vi "PicoScope2000aExampleBlockMSO.vi"() -> ()   [LabVIEW 2010]
doc: "ps2000a API Block Capture example"
uses:
  shared/PicoBuffers.ctl
  <vilib>/Waveform/DWDTOps.llb/DWDT Analog to Digital.vi
  shared/Buffer and Transfer Settings.ctl
  shared/Acquisition Settings.ctl
  PicoScope2000aLib/PicoScope2000aAnalogChannelSettings.ctl
  PicoScope2000aLib/PicoScope2000aDigitalChannelSettings.ctl
panel:
  out "Pico 2000a Units":string
  in  "roundFaster":bool=TRUE
  in  "timeIntervalRequested":dbl format="%#6_6p"
  in  "Write to TDMS":bool
  out "Properties Panel":T1 {"Max Total Capture Time Available (sec)" format="%.3p"; "Sample Frequency" format="%.3p"; "Sample Internal" format="%.3p"; "Max Samples Available" format="%.3p"; "Total Capture Time (sec)" format="%.3p"}
  in  "Port 0 Settings":T2={"Enabled"=FALSE, "Logic Level"=9830} {"Logic Level" items=["1.5V TTL"=9830, "2.5V CMOS"=16383]}
  in  "Channel A Settings":T3={"Enabled"=TRUE, "Coupling"=1, "Range"=6, "Analogue Offset"=0.0} {"Analogue Offset" format="%#_6p"; "Range" items=["20 mV"=1, "50 mV"=2, "100 mV"=3, "200 mV"=4, "500 mV"=5, "1 V"=6, "2 V"=7, "5 V"=8, "10 V"=9, "20 V"=10]; "Coupling" items=["AC", "DC"]}
  out "Device Info":T4={"Driver Version"="0", "USB Version"="0", "Hardware"="1", "Variant"="0", "Batch and Serial"="0", "Cal Date"="0", "Kernel Version"="0", "Digital HW Version"="0", "Analogue HW Version"="0", "Firmware 1"="0", "Firmware 2"="0", "MSO"=FALSE, "Number of Channels"=0}
  out "overflow":i16 format="%06b"
  in  "Apply Settings":bool
  in  "Trigger Settings":T5={"Trigger Enabled"=FALSE, "Trigger Source"=enum."Channel A", "Trigger Threshold (volts)"=0.0, "Trigger Direction"=2, "Trigger Delay (samples)"=0, "Auto Trigger Time (ms)"=1000} {"Trigger Direction" items=["Rising"=2, "Falling"=3]}
  out "error out":errorcluster
  in  "Data file":path=path "PicoScope2000aExampleBlock Data"
  in  "Buffer and Transfer Settings":T6={"startIndex"=0, "Samples"=32000, "Down Sample Ratio"=1, "Down-Sample Mode"=0} {"Down-Sample Mode" items=["RAW none"=2147483648, "None"=0, "Aggregate"=1, "Decimate"=2, "Average"=4]; "Down Sample Ratio" step=1; "Samples" format="%_6p"}
  in  "Acquisition Settings":T7={"preTriggerSamples"=0, "postTriggerSamples"=32000, "timebase"=0} {"postTriggerSamples" format="%_6p"; "preTriggerSamples" format="%_6p"}
  out "Port 0":digitalwaveform(graph)={"t0"=timestamp(0 s since 1904-01-01), "dt"=8e-09, "Y"={"transitions"=[], "data"=[]}}
  in  "stop":bool
  out "Analog Channels":cluster{i32, sgl, "Data":dbl[]}[](graph)
  in  "Serial Number":string
  in  "Use Serial Number":bool
  in  "error in (no error)":errorcluster
  # "Bit 0 = ChA"
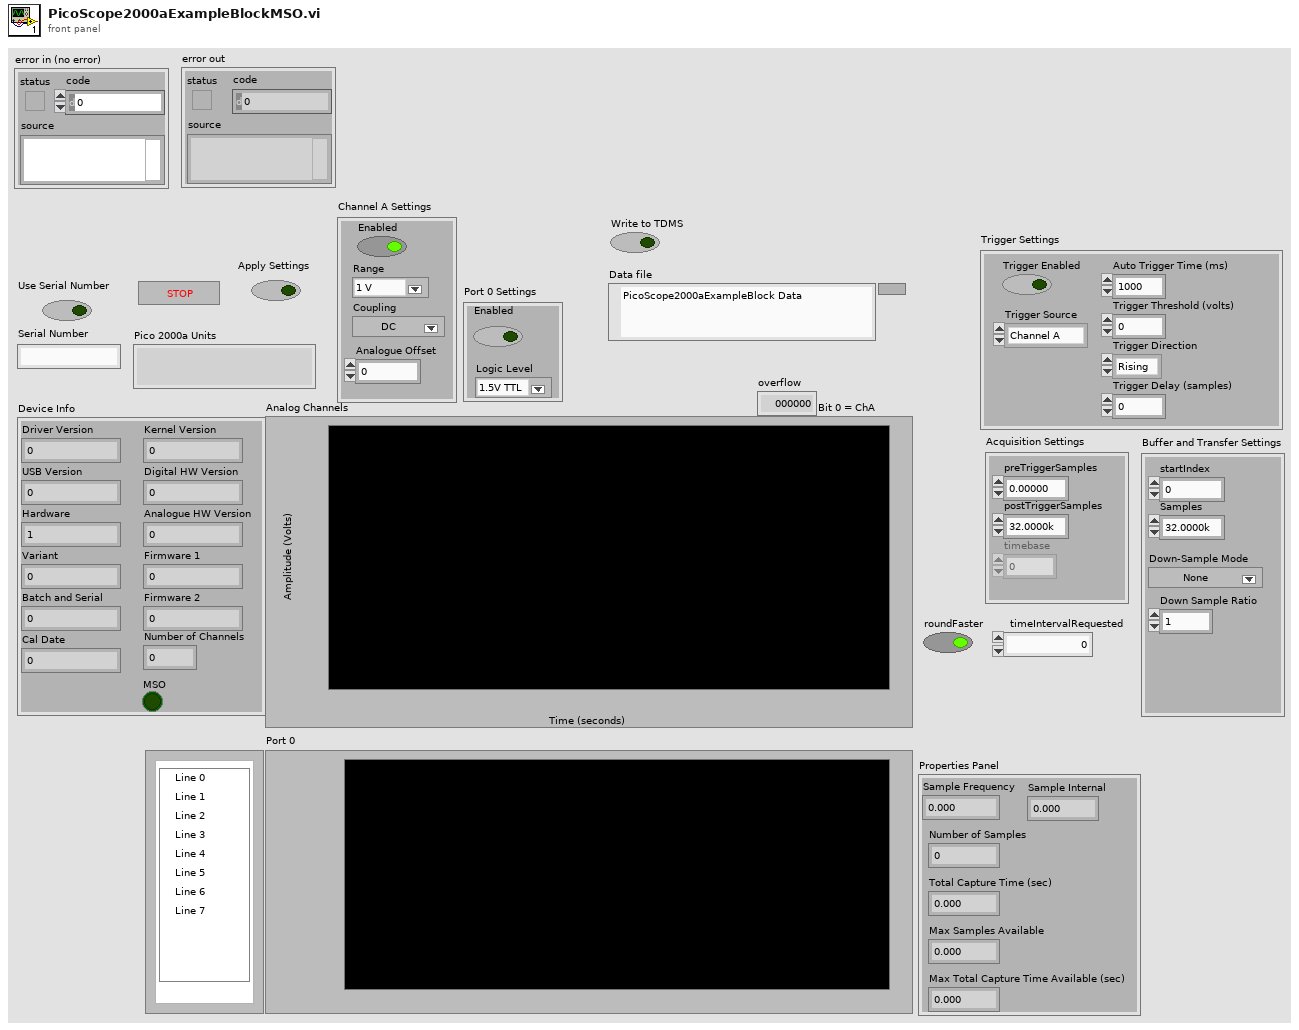
[diagram p1: front panel]
types:
  T1 = cluster{"Sample Frequency":sgl, "Sample Internal":sgl, "Max Samples Available":i32, "Number of Samples":u32, "Total Capture Time (sec) ":sgl, "Max Total Capture Time Available (sec)":sgl}
  T2 = typedef "PicoScope2000aDigitalChannelSettings.ctl" = cluster{"Enabled":bool, "Logic Level":i16}
  T3 = typedef "PicoScope2000aAnalogChannelSettings.ctl" = cluster{"Enabled":bool, "Coupling":i16, "Range":u32, "Analogue Offset":sgl}
  T4 = cluster{"Driver Version":string, "USB Version":string, "Hardware":string, "Variant":string, "Batch and Serial":string, "Cal Date":string, "Kernel Version":string, "Digital HW Version":string, "Analogue HW Version":string, "Firmware 1":string, "Firmware 2":string, "MSO":bool, "Number of Channels":i16}
  T5 = cluster{"Trigger Enabled":bool, "Trigger Source":enum16{"Channel A", "Channel B", "Channel C", "Channel D", "Ext."}, "Trigger Threshold (volts)":dbl, "Trigger Direction":u16, "Trigger Delay (samples)":u32, "Auto Trigger Time (ms)":i16}
  T6 = typedef "Buffer and Transfer Settings.ctl" = cluster{"startIndex":u64, "Samples":u64, "Down Sample Ratio":u64, "Down-Sample Mode":u32}
  T7 = typedef "Acquisition Settings.ctl" = cluster{"preTriggerSamples":u64, "postTriggerSamples":u64, "timebase":u32}
  T8 = typedef "PicoBuffers.ctl" = cluster{"Max Buffer Pointers":u64[][][], "Min Buffer Pointers":u64[][][], "StreamingDataInfo":cluster{"Channel":u32, "Down-Sample Mode":u32, "PICO_DATA_TYPE":enum32{"PICO_INT8_T", "PICO_INT16_T", "PICO_INT32_T", "PICO_UINT32_T", "PICO_INT64_T", ""}, "Samples":i32, "bufferIndex":u64, "startIndex":i32, "overflow":i16}[][]}
  T9 = enum16{"open", "open or create", "create or replace", "create", "open (read-only)"}
  T10 = cluster{"Channel A Buffer":i16[], "Channel B Buffer":i16[], "Channel C Buffer":i16[], "Channel D Buffer":i16[], "Channel E Buffer":i16[], "Channel F Buffer":i16[], "Channel G Buffer":i16[], "Channel H Buffer":i16[], "Port 0 Buffer":i16[], "Port 1 Buffer":i16[]}[]
  T11 = cluster{"Channel A Buffer":i16[], "Channel B Buffer":i16[], "Channel C Buffer":i16[], "Channel D Buffer":i16[], "Channel E Buffer":i16[], "Channel F Buffer":i16[], "Channel G Buffer":i16[], "Channel H Buffer":i16[], "Port 0 Buffer":i16[], "Port 1 Buffer":i16[]}
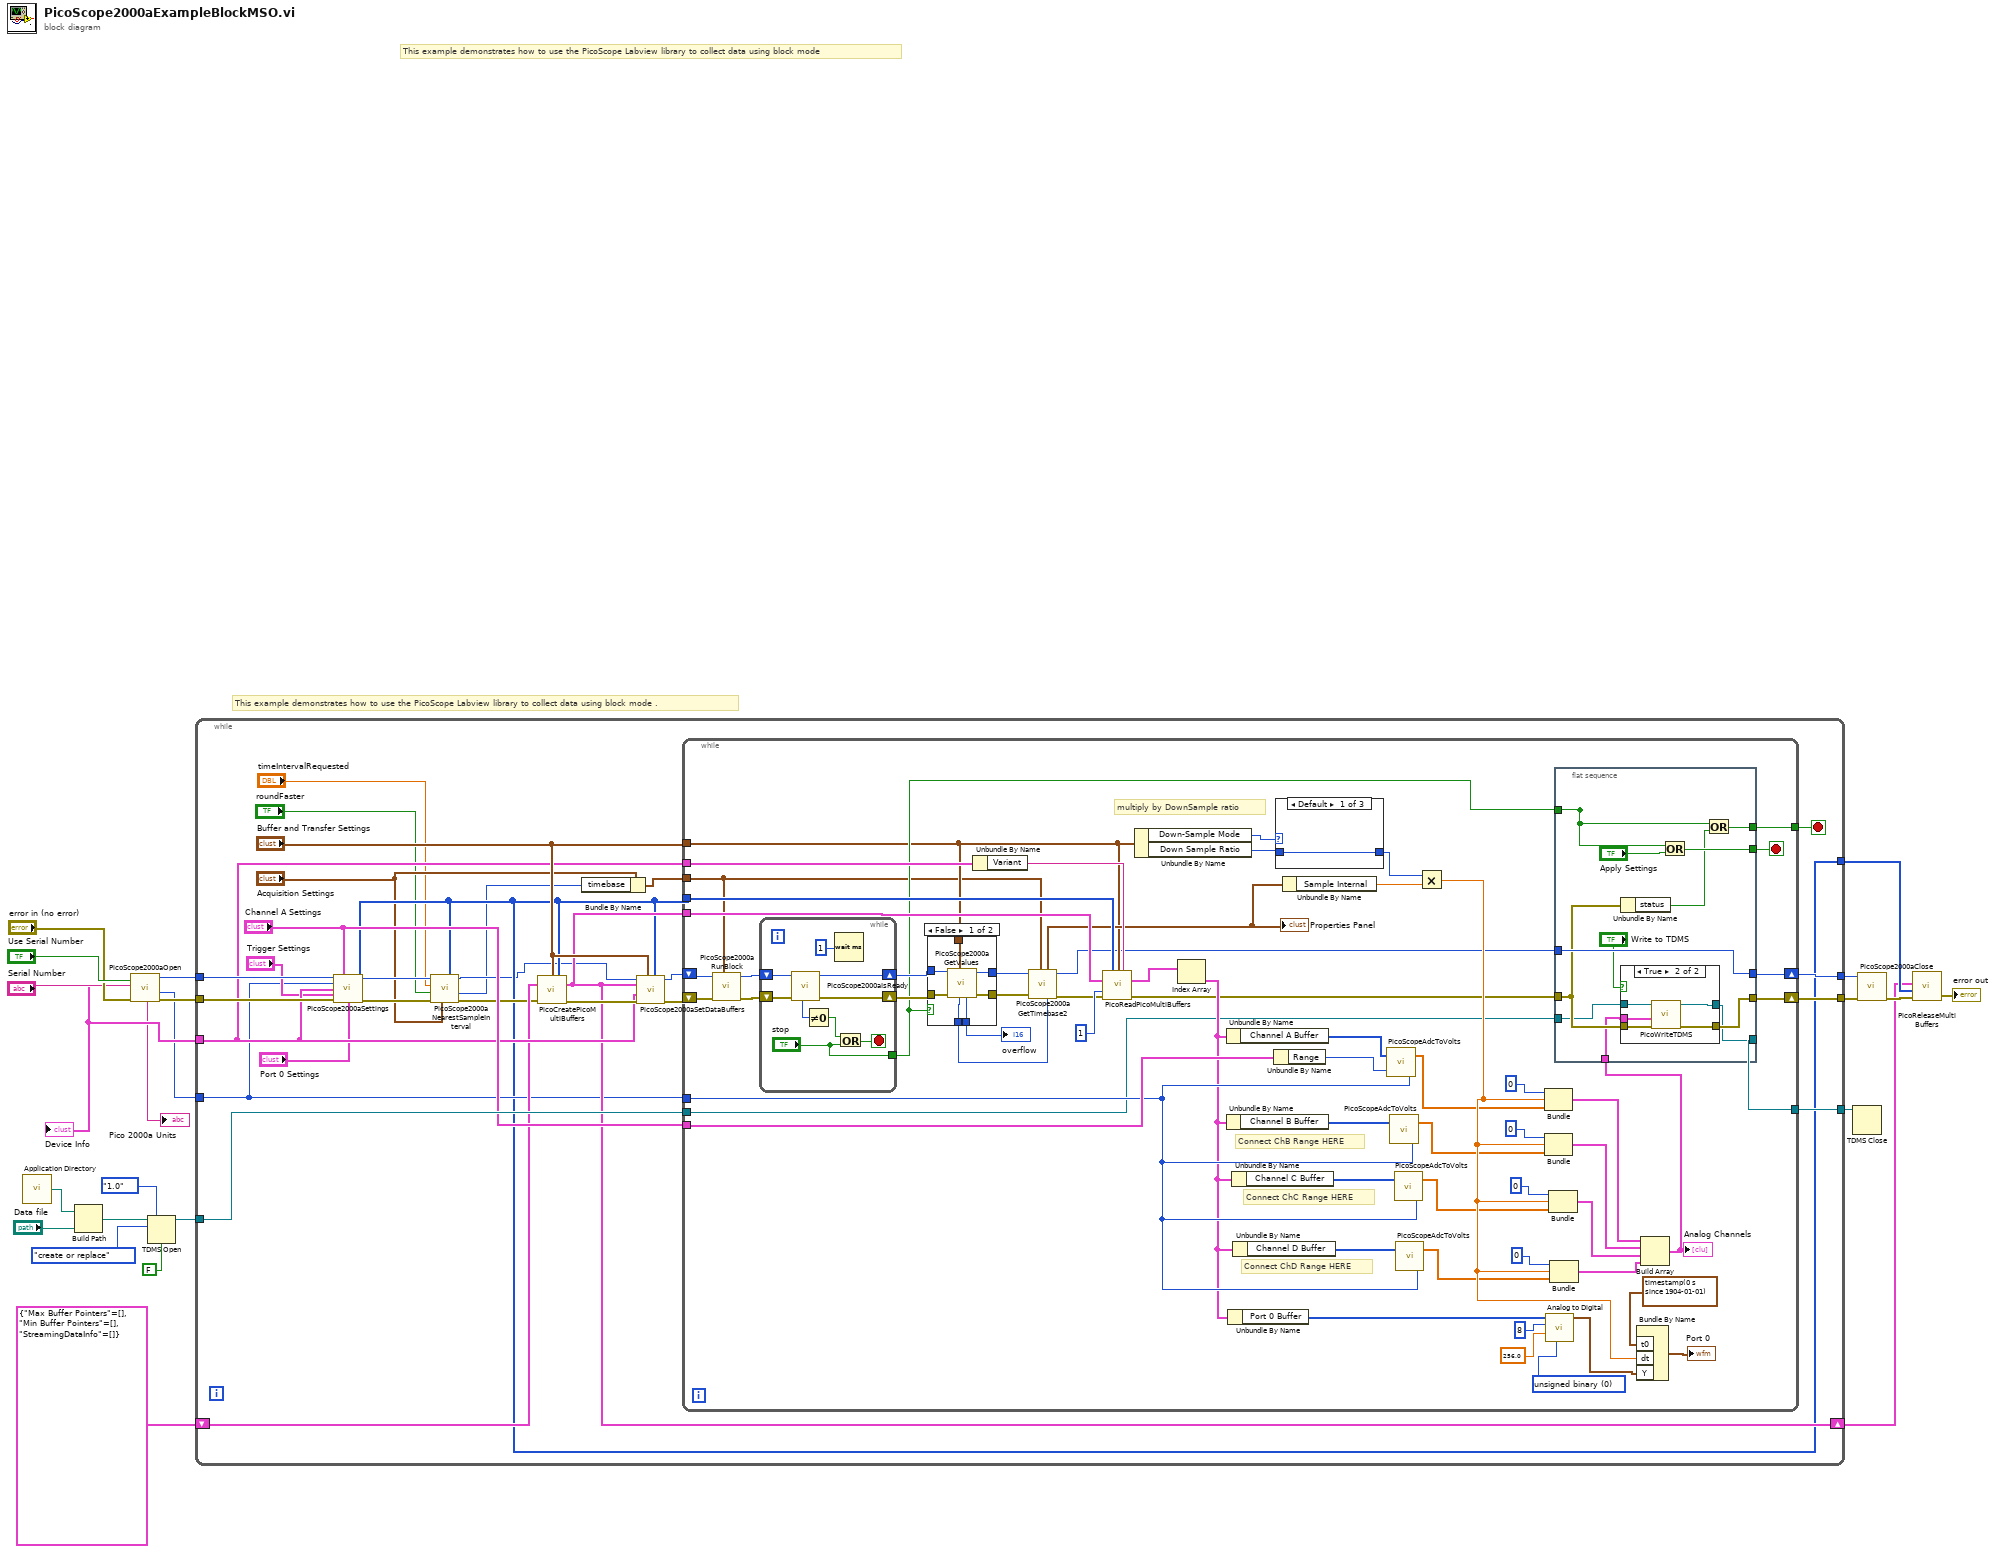
[diagram p0: block diagram]
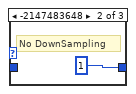
[diagram p4: hidden frame]
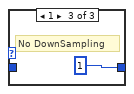
[diagram p5: hidden frame]
diagram:
  # "This example demonstrates how to use the PicoScope Labview library to collect data using block mode ."
  # "This example demonstrates how to use the PicoScope Labview library to collect data using block mode"
  n1 = call <vilib>:"Application Directory.vi"() -> ("Application Directory"=w16:path)
  n2 = Build Path(base path=w16, name or relative path="Data file") -> (appended path=w17:path)
  n3 = call "PicoScope2000aOpen.vi"("Serial Number"="Serial Number", "Use Serial Number"="Use Serial Number", "error in (no error)"="error in (no error)") -> ("error out"=w9:errorcluster, "Max Adc value"=w4:i16, "Device Info"=w7:T4, "handle"=w23:i16, "Pico 2000a Units"=→"Pico 2000a Units":string)  [unwired: 3 in, 1 out]
  "Device Info" <- w7
  n4 = TDMS Open(6:FALSE ("disable buffering? (T)"), 7:enum16{"1.0", "2.0"}."1.0" ("file format version (2.0)"), 10:T9."create or replace" ("operation (0:open)"), 11:w17) -> (3:w14:refnum<k34>)  [unwired: 2 in, 1 out]
  n5 = while {
    tunnel: w23 -> [w41]
    tunnel: w4 -> [w34]
    tunnel: [w30] -> w22
    tunnel: [w48] -> w15
    tunnel: w14 -> [w50]
    tunnel: w7 -> [w39]
    tunnel: w9 -> [w40]
    tunnel: [w49] -> w6
    tunnel: [w46] -> w8
    shift-right: [w36] -> w2
    shift-left: T8 {"Max Buffer Pointers"=[], "Min Buffer Pointers"=[], "StreamingDataInfo"=[]} ("Data Pointers") -> [w35]
    stop <- w47 stop-if-true
    n6 = call "PicoScope2000aSettings.vi"("handle in"=w41, "Channel A Settings"="Channel A Settings", "Max_adc"=w34, "Device Info"=w39, "Trigger Settings"="Trigger Settings", "error in"=w40, "Port 0 Settings"="Port 0 Settings") -> ("handle out"=w31:i16, "Enabled Array"=w30:i16[], "error out"=w33:errorcluster)  [unwired: 6 in]
    n7 = call "PicoScope2000aNearestSampleInterval.vi"("Enabled array"=w30, "Acquisition Settings"="Acquisition Settings", "error in (no error)"=w33, "roundFaster"="roundFaster", "timeIntervalRequested"="timeIntervalRequested", "handle in"=w31) -> ("error out"=w32:errorcluster, "timebase"=w27:u32, "handle out"=w29:i16)  [unwired: 2 in, 1 out]
    n8 = call "PicoCreatePicoMultiBuffers.vi"("Buffer and Transfer Settings"="Buffer and Transfer Settings", "enabled array"=w30, "Data Pointers In"=w35, "error in (no error)"=w32) -> ("Data Pointers"=w36:T8, "error out"=w51:errorcluster)  [unwired: 10 in]
    n9 = Bundle By Name(cluster="Acquisition Settings", "timebase"=w27) -> (w24:T7)
    n10 = call "PicoScope2000aSetDataBuffers.vi"("enabled array"=w30, "Buffer and Transfer Settings"="Buffer and Transfer Settings", "error in (no error)"=w51, "Device Info"=w39, "Data Pointers In"=w36, "handle in"=w29) -> ("error out"=w45:errorcluster, "handle out"=w44:i16)  [unwired: 4 in]
    n11 = while {
      tunnel: w36 -> [w113]
      tunnel: "Buffer and Transfer Settings" -> [w60]
      tunnel: w30 -> [w105]
      tunnel: "Channel A Settings" -> [w104]
      tunnel: w24 -> [w59]
      tunnel: w34 -> [w103]
      tunnel: w39 -> [w100]
      tunnel: [w71] -> w47
      shift-right: [w73] -> w49
      shift-left: w45 -> [w65]
      shift-right: [w69] -> w46
      shift-left: w44 -> [w66]
      tunnel: w50 -> [w54]
      tunnel: [w52] -> w48
      stop <- w70 stop-if-true
      w90 = u16 0 items=["unsigned binary", "offset binary", "2's complement"] ("data format (offset binary)")
      # "Connect ChB Range HERE"
      # "Connect ChD Range HERE"
      # "Connect ChC Range HERE"
      # "multiply by DownSample ratio"
      n12 = call "PicoScope2000aRunBlock.vi"("Acquisition Settings"=w59, "error in (no error)"=w65, "handle in"=w66) -> ("error out"=w107:errorcluster, "handle out"=w106:i16)  [unwired: 5 in, 2 out]
      n13 = while {
        shift-right: [w149] -> w67
        shift-left: w107 -> [w150]
        shift-right: [w148] -> w68
        shift-left: w106 -> [w147]
        tunnel: ["stop"] -> w64
        stop <- w144 stop-if-true
        n14 = call "PicoScope2000aIsReady.vi"("error in (no error)"=w150, "handle in"=w147) -> ("error out"=w149:errorcluster, "handle out"=w148:i16, "ready"=w146:i16)  [unwired: 7 in]
        n15 = Not Equal To 0?(x=w146) -> (x != 0?=w145:bool)
        n16 = Wait (ms)(milliseconds to wait=u32 1) -> ()  [unwired: 1 out]
        n17 = Or(x=w145, y="stop") -> (x .or. y?=w144:bool)
      }
      n18 = case shown="False" w64 {
        tunnel: w67 -> [w120 w121]
        tunnel: w68 -> [w119 w122]
        tunnel: [w118 w122] -> w57
        tunnel: [w117 w121] -> w58
        tunnel: w60 -> [w116 _]
        tunnel: [w115 _] -> w63
        tunnel: [w114 _] -> w62
        frame False {
          n19 = call "PicoScope2000aGetValues.vi"("Buffer and Transfer Settings"=w116, "error in (no error)"=w120, "handle in"=w119) -> ("error out"=w117:errorcluster, "handle out"=w118:i16, "overflow"=w115:i16, "noOfSamples"=w114:u64)  [unwired: 5 in]
        }
        frame True {
        }
      }
      "overflow" <- w63
      n20 = Unbundle By Name(w100) -> ("Variant"=w101:string)
      n21 = call "PicoScope2000aGetTimebase2.vi"("Number of Samples"=w62, "Acquisition Settings"=w59, "error in (no error)"=w58, "handle in"=w57) -> ("error out"=w56:errorcluster, "handle out"=w55:i16, "Properties Panel"=w61:T1)  [unwired: 5 in]
      "Properties Panel" <- w61
      n22 = call "PicoReadPicoMultiBuffers.vi"("enabled array"=w105, "Buffer and Transfer Settings"=w60, "Variant"=w101, "Data Pointers"=w113, "No of Buffers"=1, "error in (no error)"=w56) -> ("MultiBuffers (Max or non-aggregated)"=w112:T10, "error out"=w72:errorcluster)  [unwired: 7 in, 1 out]
      n23 = Unbundle By Name(w60) -> ("Down-Sample Mode"=w110:u32, "Down Sample Ratio"=w111:u64)
      n24 = Index Array(array=w112) -> (element=w74:T11)  [unwired: 1 in]
      n25 = Unbundle By Name(w74) -> ("Channel A Buffer"=w83:i16[])
      n26 = Unbundle By Name(w74) -> ("Channel B Buffer"=w95:i16[])
      n27 = Unbundle By Name(w74) -> ("Port 0 Buffer"=w88:i16[])
      n28 = Unbundle By Name(w74) -> ("Channel C Buffer"=w81:i16[])
      n29 = Unbundle By Name(w74) -> ("Channel D Buffer"=w77:i16[])
      n30 = Unbundle By Name(w104) -> ("Range"=w97:u32)
      n31 = case shown="Default" w110 {
        tunnel: [w151 u64 1 ("Down Sample Ratio") u64 1 ("Down Sample Ratio")] -> w108
        tunnel: w111 -> [w151 _ _]
        frame Default {
        }
        frame -2147483648 {
          # "No DownSampling"
        }
        frame 1 {
          # "No DownSampling"
        }
      }
      n32 = Unbundle By Name(w61) -> ("Sample Internal"=w102:sgl)
      n33 = call "PicoScopeAdcToVolts.vi"("Max_adc"=w103, "Range Index"=w97, "Data"=w83) -> ("Data"=w84:dbl[])
      n34 = call "PicoScopeAdcToVolts.vi"("Max_adc"=w103, "Data"=w95) -> ("Data"=w94:dbl[])  [unwired: 1 in]
      n35 = call "PicoScopeAdcToVolts.vi"("Max_adc"=w103, "Data"=w81) -> ("Data"=w80:dbl[])  [unwired: 1 in]
      n36 = call "PicoScopeAdcToVolts.vi"("Max_adc"=w103, "Data"=w77) -> ("Data"=w76:dbl[])  [unwired: 1 in]
      n37 = Multiply(x=w108, y=w102) -> (x*y=w109:sgl)
      n38 = Bundle(0, w109, "Data"=w84) -> (w93:cluster{i32, sgl, "Data":dbl[]})  [unwired: 1 in]
      n39 = Bundle(0, w109, "Data"=w94) -> (w92:cluster{i32, sgl, "Data":dbl[]})  [unwired: 1 in]
      n40 = call-poly <vilib>:"Analog to Digital.vi"("data format (offset binary)"=w90, "full-scale range (pk-pk)"=256.0, "resolution (16 bit)"=8, "analog waveform"=w88) -> ("digital waveform"=w85:digitalwaveform)  [unwired: 4 in, 3 out]
      n41 = Bundle(0, w109, "Data"=w80) -> (w79:cluster{i32, sgl, "Data":dbl[]})  [unwired: 1 in]
      n42 = Bundle(0, w109, "Data"=w76) -> (w75:cluster{i32, sgl, "Data":dbl[]})  [unwired: 1 in]
      n43 = flat-sequence {
        tunnel: [w134] -> w70
        tunnel: [w129] -> _
        tunnel: [w131] -> w71
        tunnel: w55 -> [w130]
        tunnel: [w130] -> w69
        tunnel: w72 -> [w128]
        tunnel: [w124] -> w73
        tunnel: w64 -> [w129]
        tunnel: w54 -> [w126]
        tunnel: w53 -> [w125]
        tunnel: [w123] -> w52
        frame #0 {
          n44 = Unbundle By Name(w128) -> ("status"=w132:bool)
          n45 = case shown="True" "Write to TDMS" {
            tunnel: w125 -> [_ w141]
            tunnel: w126 -> [w135 w140]
            tunnel: w128 -> [w136 w139]
            tunnel: [w136 w138] -> w124
            tunnel: [w135 w137] -> w123
            frame False {
            }
            frame True {
              n46 = call "PicoWriteTDMS.vi"("error in (no error)"=w139, "Analog Channels"=w141, "Refnum in"=w140) -> ("error out"=w138:errorcluster, "Refnum out"=w137:refnum<k34>)  [unwired: 7 in]
            }
          }
          n47 = Or(x=w129, y="Apply Settings") -> (x .or. y?=w134:bool)
          n48 = Or(x=w129, y=w132) -> (x .or. y?=w131:bool)
        }
      }
      n49 = Bundle By Name("t0"=timestamp(0 s since 1904-01-01), "dt"=w109, "Y"=w85) -> (→"Port 0":digitalwaveform)  [unwired: 1 in]
      n50 = Build Array(w93, w92, w79, w75) -> (w53:cluster{i32, sgl, "Data":dbl[]}[])
      "Analog Channels" <- w53
    }
  }
  n51 = TDMS Close(11:w15) -> ()  [unwired: 1 in, 2 out]
  n52 = call "PicoScope2000aClose.vi"("error in (no error)"=w6, "handle in"=w8) -> ("error out"=w5:errorcluster)  [unwired: 8 in, 1 out]
  n53 = call "PicoReleaseMultiBuffers.vi"("error in (no error)"=w5, "Enabled array"=w22, "Data Pointers"=w2) -> ("error out"=→"error out":errorcluster)  [unwired: 7 in, 1 out]
